vi "New Node On Wire_CLEANUP.vi"(8 "error in":errorcluster, 11 "Temporary Node":refnum<vi>) -> (0 "error out":errorcluster)   [LabVIEW 2023]
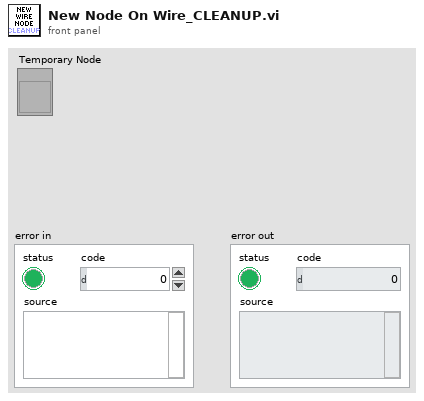
[diagram p1: front panel]
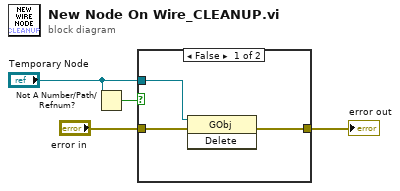
[diagram p0: block diagram]
diagram:
  n1 = Not A Number/Path/Refnum?(number/path/refnum="Temporary Node") -> (NaN/Path/Refnum?=w1:bool)
  n2 = case shown="False" w1 {
    tunnel: "Temporary Node" -> [w7 _]
    tunnel: "error in" -> [w6 w8]
    tunnel: [w5 w8] -> w3
    frame False {
      n3 = invoke class="GObj" method="Delete"(reference=w7, error in=w6) -> (error out=w5:errorcluster)  [unwired: 1 in, 2 out]
    }
    frame True {
    }
  }
  "error out" <- w3
